vi "Hardware Interface.vi"(11 "message queue":refnum<queue>) -> ()   [LabVIEW 2026]
uses:
  Queue Data.ctl
panel:
  in  "Broken Arrow":bool
  in  "Spaghetti":bool
  in  "Fixed Bug":bool
  in  "Sleep":bool
  in  "Clean":bool
  in  "stop":bool
  in  "Feed":bool
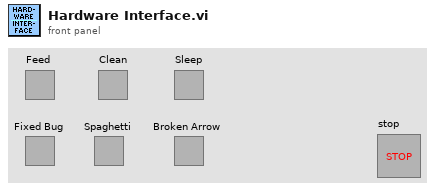
[diagram p1: front panel]
types:
  T1 = typedef "Queue Data.ctl" = cluster{"State":string, "Data":variant}
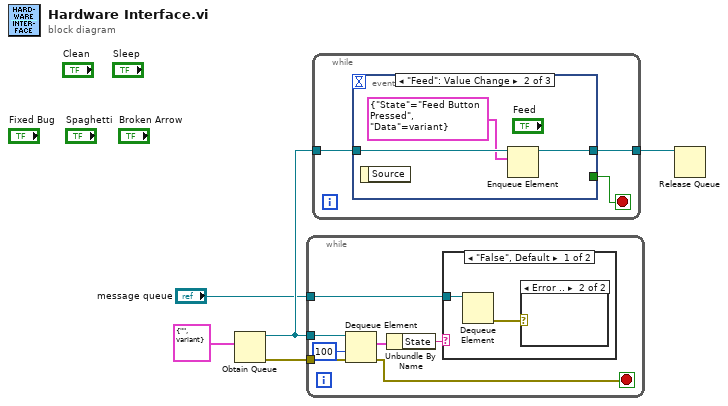
[diagram p0: block diagram]
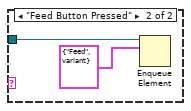
[diagram p3: hidden frame]
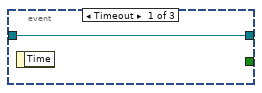
[diagram p4: hidden frame]
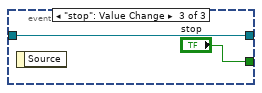
[diagram p5: hidden frame]
diagram:
  n1 = Obtain Queue(element data type=T1 {"State"="", "Data"=variant} ("Queue Data")) -> (queue out=w3:refnum<queue>, error out=w4:errorcluster)  [unwired: 4 in, 1 out]
  n2 = while {
    tunnel: w4 -> [w12]
    tunnel: w3 -> [w11]
    tunnel: "message queue" -> [w7]
    stop <- w10 stop-if-true
    n3 = Dequeue Element(queue=w11, timeout in ms (-1)=100, error in (no error)=w12) -> (element=w9:T1, error out=w10:errorcluster)  [unwired: 2 out]
    n4 = Unbundle By Name(w9) -> ("State"=w8:string)
    n5 = case shown="\"False\", Default" w8 {
      tunnel: w7 -> [w14 w16]
      frame "False", Default {
        n6 = Dequeue Element(queue=w14) -> (error out=w13:errorcluster)  [unwired: 2 in, 3 out]
        n7 = case shown="Error .." w13 {
          frame No Error {
          }
          frame Error {
          }
        }
      }
      frame "Feed Button Pressed" {
        n8 = Enqueue Element(queue=w16, element=T1 {"State"="Feed", "Data"=variant}) -> ()  [unwired: 2 in, 3 out]
      }
    }
  }
  n9 = while {
    tunnel: w3 -> [w18]
    tunnel: [w17] -> w2
    stop <- w19 stop-if-true
    n10 = event shown="[1] \"Feed\": Value Change" {
      selector: _ -> [_ _ _]
      dyn-events: _ -> [_ _ _]
      timeout: _ -> [_ _ _]
      tunnel: [_ _ "stop"] -> w19
      tunnel: w18 -> [w20 w23 w24]
      tunnel: [w20 w22 w24] -> w17
      event Timeout {
        n11 = event-data() -> ()  [unwired: 1 in, 1 out]
      }
      event "Feed": Value Change {
        n12 = event-data() -> ()  [unwired: 1 in, 1 out]
        n13 = Enqueue Element(queue=w23, element=T1 {"State"="Feed Button Pressed", "Data"=variant}) -> (queue out=w22:refnum<queue>)  [unwired: 2 in, 2 out]
      }
      event "stop": Value Change {
        n14 = event-data() -> ()  [unwired: 1 in, 1 out]
      }
    }
  }
  n15 = Release Queue(queue=w2) -> ()  [unwired: 2 in, 3 out]
